vi "DOTNET - Network Ping v2.0.vi"(0 "IP/Address":string="127.0.0.1", 5 "SetSize":i32=32, 7 "timeout":i32=100, 11 "error in (no error)":errorcluster) -> (4 "Status":i32(ring) items=["Success"=0, "DestinationNetworkUnreachable"=11002, "DestinationHostUnreachable"=11003, "DestinationProhibited, DestinationProtocolUnreachable"=11004, "DestinationPortUnreachable"=11005, "NoResources"=11006, "BadOption"=11007, "HardwareError"=11008, "PacketTooBig"=11009, "TimedOut"=11010, "BadRoute"=11012, "TtlExpired"=11013, "TtlReassemblyTimeExceeded"=11014, "ParameterProblem"=11015, "SourceQuench"=11016, "BadDestination"=11018, "DestinationUnreachable"=11040, "TimeExceeded"=11041, "BadHeader"=11042, "UnrecognizedNextHeader"=11043, "IcmpError"=11044, "DestinationScopeMismatch"=11045, "Unknown"=-1], 6 "RoundtripTime":i64, 15 "error out":errorcluster)   [LabVIEW 2019]
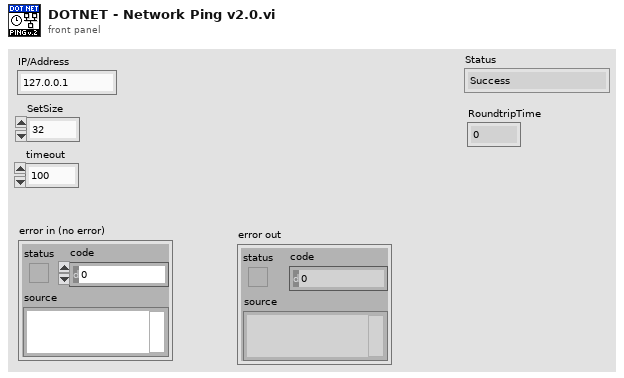
[diagram p1: front panel]
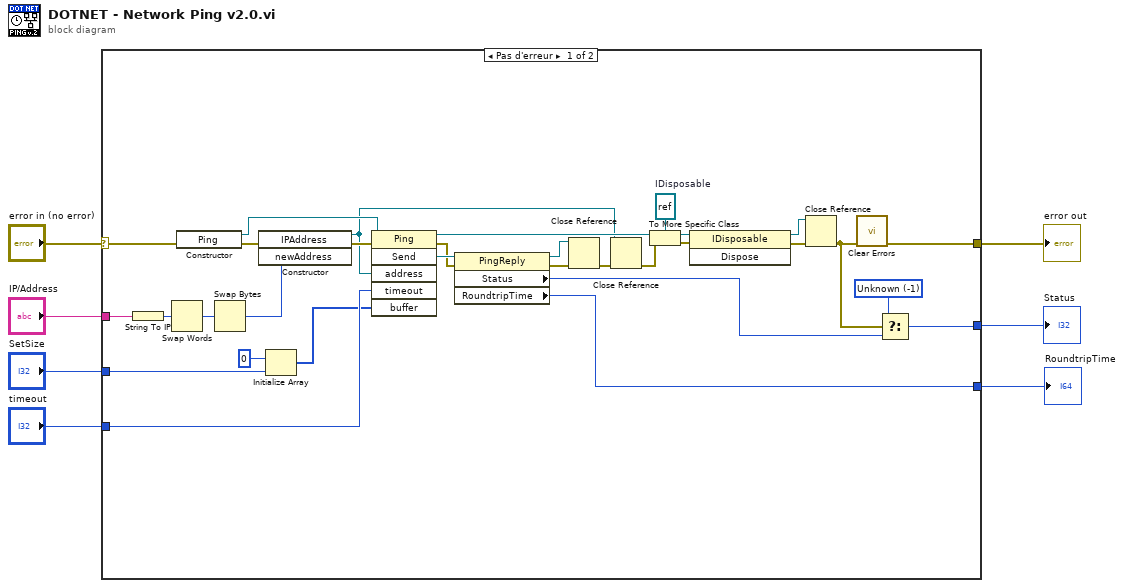
[diagram p0: block diagram]
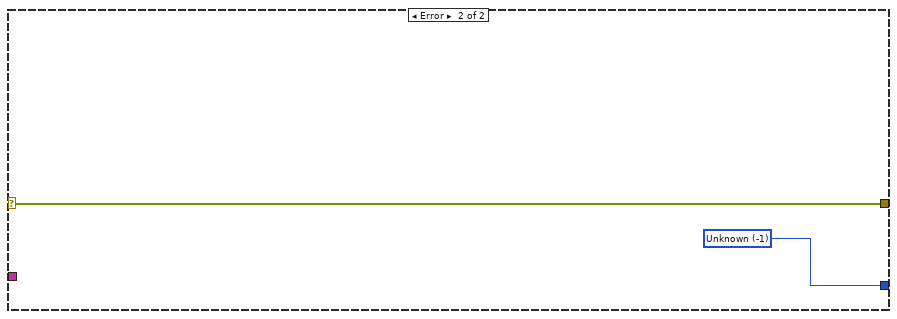
[diagram p2: hidden frame]
diagram:
  n1 = case shown="Pas d'erreur" "error in (no error)" {
    selector: "error in (no error)" -> [w12 w40]
    tunnel: "IP/Address" -> [w38 _]
    tunnel: "timeout" -> [w37 _]
    tunnel: "SetSize" -> [w36 _]
    tunnel: [w9 w39] -> w4
    tunnel: [w35 _] -> w3
    tunnel: [w34 w40] -> w2
    frame No Error {
      w8 = -1 items=["Success"=0, "DestinationNetworkUnreachable"=11002, "DestinationHostUnreachable"=11003, "DestinationProhibited, DestinationProtocolUnreachable"=11004, "DestinationPortUnreachable"=11005, "NoResources"=11006, "BadOption"=11007, "HardwareError"=11008, "PacketTooBig"=11009, "TimedOut"=11010, "BadRoute"=11012, "TtlExpired"=11013, "TtlReassemblyTimeExceeded"=11014, "ParameterProblem"=11015, "SourceQuench"=11016, "BadDestination"=11018, "DestinationUnreachable"=11040, "TimeExceeded"=11041, "BadHeader"=11042, "UnrecognizedNextHeader"=11043, "IcmpError"=11044, "DestinationScopeMismatch"=11045, "Unknown"=-1] ("Status")
      w22 = refnum<k24> refnum  # IDisposable
      n2 = String To IP(1:w38) -> (0:w26:u32)
      n3 = Swap Words(1:w26) -> (0:w24:u32)
      n4 = constructor class="Ping"(error in=w12) -> (reference out=w31:refnum<k24>, error out=w28:errorcluster)  [unwired: 2 in, 1 out]
      n5 = Swap Bytes(anything=w24) -> (byte swapped=w25:u32)
      n6 = constructor class="IPAddress"(error in=w28, "newAddress"=w25) -> (reference out=w18:refnum<k24>, error out=w27:errorcluster)  [unwired: 2 in, 2 out]
      n7 = Initialize Array(u8 0, w36) -> (w30:u8[])
      n8 = invoke class="Ping" method="Send"(reference=w31, error in=w27, "address"=w18, "timeout"=w37, "buffer"=w30) -> (reference out=w23:refnum<k24>, error out=w32:errorcluster, "Send"=w33:refnum<k24>)  [unwired: 1 in, 3 out]
      n9 = property class="PingReply"(reference=w33, error in=w32) -> (reference out=w21:refnum<k24>, error out=w20:errorcluster, "Status"=w10:i32, "RoundtripTime"=w35:i64)
      n10 = Close Reference(reference=w21, error in (no error)=w20) -> (error out=w19:errorcluster)
      n11 = Close Reference(reference=w18, error in (no error)=w19) -> (error out=w17:errorcluster)
      n12 = To More Specific Class(target class=w22, reference=w23, error in=w17) -> (specific class reference=w16:refnum<k24>, error out=w15:errorcluster)
      n13 = invoke class="IDisposable" method="Dispose"(reference=w16, error in=w15) -> (reference out=w13:refnum<k24>, error out=w14:errorcluster)  [unwired: 1 in, 1 out]
      n14 = Close Reference(reference=w13, error in (no error)=w14) -> (error out=w11:errorcluster)
      n15 = call <vilib>:"Clear Errors.vi"("error in (no error)"=w11) -> ("error out"=w34:errorcluster)  [unwired: 5 in, 1 out]
      n16 = Select(t=w8, s=w11, f=w10) -> (s? t:f=w9:i32)
    }
    frame Error {
      w39 = -1 items=["Success"=0, "DestinationNetworkUnreachable"=11002, "DestinationHostUnreachable"=11003, "DestinationProhibited, DestinationProtocolUnreachable"=11004, "DestinationPortUnreachable"=11005, "NoResources"=11006, "BadOption"=11007, "HardwareError"=11008, "PacketTooBig"=11009, "TimedOut"=11010, "BadRoute"=11012, "TtlExpired"=11013, "TtlReassemblyTimeExceeded"=11014, "ParameterProblem"=11015, "SourceQuench"=11016, "BadDestination"=11018, "DestinationUnreachable"=11040, "TimeExceeded"=11041, "BadHeader"=11042, "UnrecognizedNextHeader"=11043, "IcmpError"=11044, "DestinationScopeMismatch"=11045, "Unknown"=-1] ("Status")
    }
  }
  "RoundtripTime" <- w3
  "error out" <- w2
  "Status" <- w4
